vi "input.vi"(8 "error in":errorcluster, 10 "input allocation":T1, 11 "module in":refnum<class "E2E Runtime (UDP).lvclass">) -> (0 "error out":errorcluster, 2 "input data":T1, 3 "module out":refnum<class "E2E Runtime (UDP).lvclass">)   [LabVIEW 2015, in "E2E Runtime (UDP).lvclass"]
doc: "Provides an interface for reading data from a module at runtime. While this interface performs no operations, a child should provide an override which may read from any open sessions, references, or interfaces."
uses:
  E2E Runtime (UDP).lvclass
  <vilib>/NI/Tag Bus/table/data table.ctl
  E2E Runtime (UDP).lvclass/E2E Runtime (UDP).ctl
  <vilib>/NI/Tag Bus/table/data table.lvlib
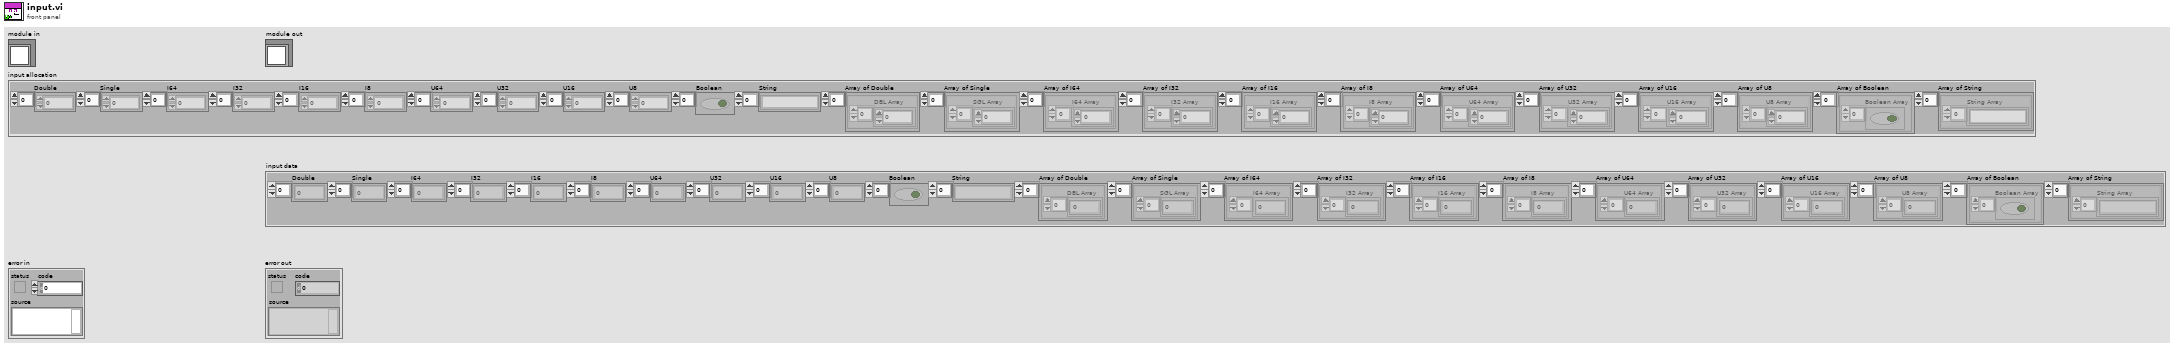
[diagram p1: front panel]
types:
  T1 = typedef "tag bus.lvlib/data table.lvlib/data table.ctl" = cluster{"Double":dbl[], "Single":sgl[], "I64":i64[], "I32":i32[], "I16":i16[], "I8":i8[], "U64":u64[], "U32":u32[], "U16":u16[], "U8":u8[], "Boolean":bool[], "String":string[], "Array of Double":cluster{"DBL Array":dbl[]}[], "Array of Single":cluster{"SGL Array":sgl[]}[], "Array of I64":cluster{"I64 Array":i64[]}[], "Array of I32":cluster{"I32 Array":i32[]}[], "Array of I16":cluster{"I16 Array":i16[]}[], "Array of I8":cluster{"I8 Array":i8[]}[], "Array of U64":cluster{"U64 Array":u64[]}[], "Array of U32":cluster{"U32 Array":u32[]}[], "Array of U16":cluster{"U16 Array":u16[]}[], "Array of U8":cluster{"U8 Array":u8[]}[], "Array of Boolean":cluster{"Boolean Array":bool[]}[], "Array of String":cluster{"String Array":string[]}[]}
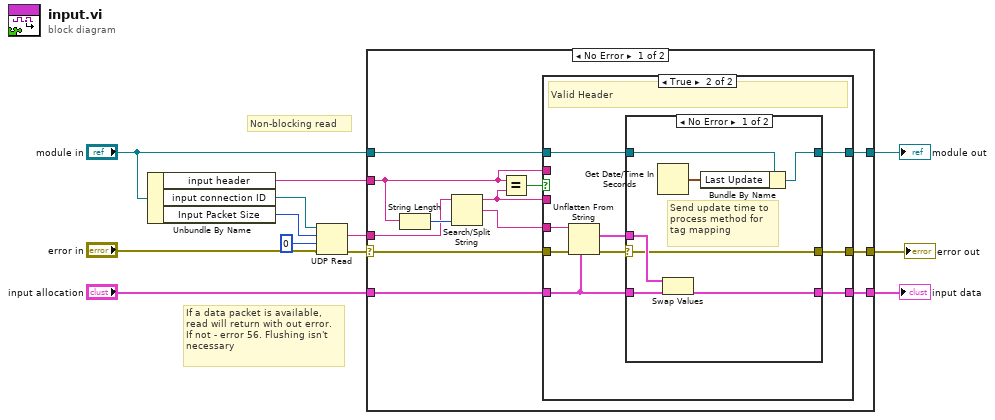
[diagram p0: block diagram]
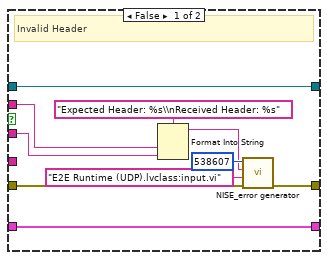
[diagram p2: hidden frame]
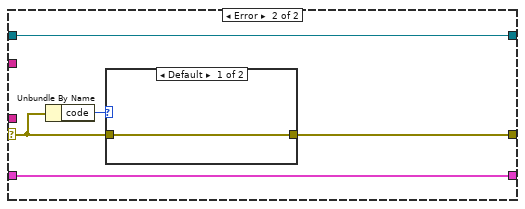
[diagram p4: hidden frame]
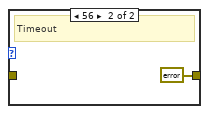
[diagram p5: hidden frame]
diagram:
  # "If a data packet is available,\nread will return with out error.\nIf not - error 56. Flushing isn't\nnecessary"
  # "Non-blocking read"
  n1 = Unbundle By Name("module in") -> ("input header"=w8:string, "input connection ID"=w11:refnum<k16>, "Input Packet Size"=w5:i32)
  n2 = UDP Read(connection ID=w11, max size (548)=w5, timeout ms (25000)=0, 8:"error in") -> (data out=w9:string, error out=w10:errorcluster)  [unwired: 3 out]
  n3 = case shown="No Error" w10 {
    selector: w10 -> [w21 w58]
    tunnel: [w15 w56] -> w1
    tunnel: w9 -> [w23 _]
    tunnel: w8 -> [w13 _]
    tunnel: "input allocation" -> [w20 w54]
    tunnel: "module in" -> [w18 w55]
    tunnel: [w17 w54] -> w3
    tunnel: [w16 w55] -> w2
    frame No Error {
      n4 = String Length(string=w13) -> (length=w24:i32)
      n5 = Search/Split String(string=w23, offset (0)=w24) -> (substring before match=w14:string, match + rest of string=w22:string)  [unwired: 1 in, 1 out]
      n6 = Equal?(x=w13, y=w14) -> (x = y?=w19:bool)
      n7 = case shown="True" w19 {
        tunnel: w22 -> [_ w43]
        tunnel: w21 -> [w32 w42]
        tunnel: w20 -> [w33 w40]
        tunnel: w18 -> [w34 w38]
        tunnel: [w33 w37] -> w17
        tunnel: [w34 w36] -> w16
        tunnel: [w31 w35] -> w15
        tunnel: w14 -> [w26 _]
        tunnel: w13 -> [w27 _]
        frame False {
          # "Invalid Header"
          n8 = Format Into String(format string="Expected Header: %s\\nReceived Header: %s", w27, w26) -> (resulting string=w25:string)  [unwired: 2 in, 1 out]
          n9 = call <vilib>:"NISE_error generator.vi"("error in"=w32, "source"="E2E Runtime (UDP).lvclass:input.vi", "append error message"=w25, "error code (0)"=538607) -> ("error out"=w31:errorcluster)  [unwired: 5 in]
        }
        frame True {
          # "Valid Header"
          n10 = Unflatten From String(type=w40, binary string=w43, error in (no error)=w42) -> (value=w41:T1, error out=w39:errorcluster)  [unwired: 2 in, 1 out]
          n11 = case shown="No Error" w39 {
            selector: w39 -> [w44 w51]
            tunnel: w41 -> [w50 _]
            tunnel: w40 -> [w49 w52]
            tunnel: w38 -> [w48 w53]
            tunnel: [w46 w52] -> w37
            tunnel: [w45 w53] -> w36
            tunnel: [w44 w51] -> w35
            frame No Error {
              # "Send update time to\nprocess method for\ntag mapping"
              n12 = Get Date/Time In Seconds() -> (seconds since 1Jan1904=w47:timestamp)
              n13 = Swap Values(12:w50, 14:w49) -> (3:w46:T1)  [unwired: 1 in, 1 out]
              n14 = Bundle By Name(cluster=w48, "Last Update"=w47) -> (w45:refnum<class "E2E Runtime (UDP).lvclass">)
            }
            frame Error {
            }
          }
        }
      }
    }
    frame Error {
      n15 = Unbundle By Name(w58) -> ("code"=w57:i32)
      n16 = case shown="Default" w57 {
        tunnel: w58 -> [w59 _]
        tunnel: [w59 errorcluster {"status"=FALSE, "code"=0, "source"=""} ("error IO")] -> w56
        frame Default {
        }
        frame 56 {
          # "Timeout"
        }
      }
    }
  }
  "error out" <- w1
  "module out" <- w2
  "input data" <- w3
